vi "PropertyChangedEventCallbackForBufferIndexDroppedFramesDiskStreamDroppedFrameAvailRam.vi"(4 "User Parameter":T1, 5 "Event Data":cluster{"sender":refnum<k24>, "e":refnum<k24>}, 6 "Control Ref":refnum<k24>, 7 "Event Common Data":T2) -> ()   [LabVIEW 2019]
uses:
  D:/SDK/PMQI-LabViewSamples/Examples/Dependencies/PVCamNET.dll
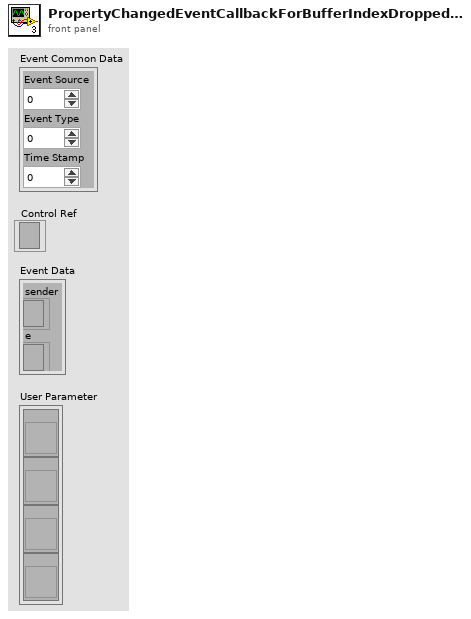
[diagram p1: front panel]
types:
  T1 = cluster{refnum<vi>, refnum<vi>, refnum<vi>, refnum<vi>}
  T2 = cluster{"Event Source":i32, "Event Type":u32, "Time Stamp":u32}
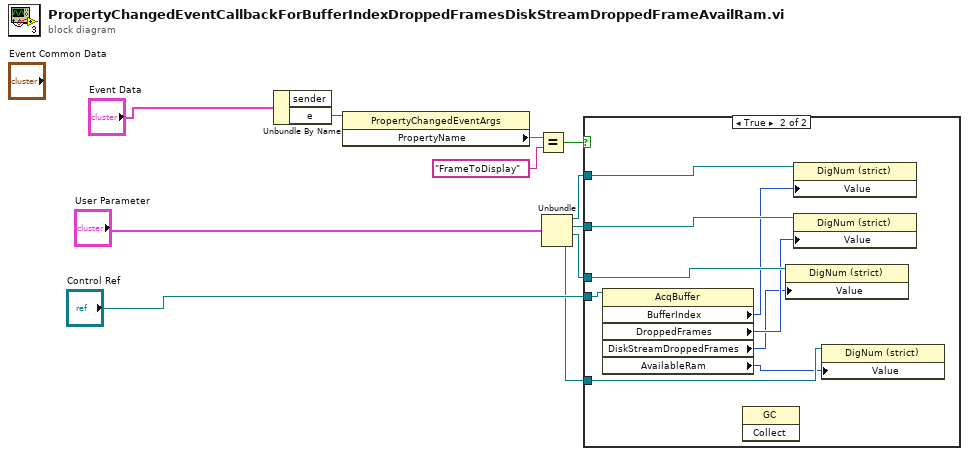
[diagram p0: block diagram]
diagram:
  n1 = Unbundle By Name("Event Data") -> ("e"=w11:refnum<k24>)  [unwired: 1 out]
  n2 = property class="PropertyChangedEventArgs"(reference=w11) -> ("PropertyName"=w10:string)  [unwired: 1 in, 2 out]
  n3 = Equal?(x=w10, y="FrameToDisplay") -> (x = y?=w8:bool)
  n4 = Unbundle("User Parameter") -> (w7:refnum<vi>, w6:refnum<vi>, w5:refnum<vi>, w1:refnum<vi>)
  n5 = case shown="True" w8 {
    tunnel: w7 -> [_ w20]
    tunnel: "Control Ref" -> [_ w19]
    tunnel: w6 -> [_ w18]
    tunnel: w5 -> [_ w17]
    tunnel: w1 -> [_ w13]
    frame False {
    }
    frame True {
      n6 = property class="AcqBuffer"(reference=w19) -> ("BufferIndex"=w16:i32, "DroppedFrames"=w15:i32, "DiskStreamDroppedFrames"=w14:u64, "AvailableRam"=w12:u64)  [unwired: 1 in, 2 out]
      n7 = invoke class="GC" method="Collect"() -> ()  [unwired: 3 in, 3 out]
      n8 = property class="DigNum (strict)"(reference=w17, "Value"=w14) -> ()  [unwired: 1 in, 2 out]
      n9 = property class="DigNum (strict)"(reference=w20, "Value"=w16) -> ()  [unwired: 1 in, 2 out]
      n10 = property class="DigNum (strict)"(reference=w18, "Value"=w15) -> ()  [unwired: 1 in, 2 out]
      n11 = property class="DigNum (strict)"(reference=w13, "Value"=w12) -> ()  [unwired: 1 in, 2 out]
    }
  }
